vi "H5Sextent_copy.vi"(6 "error in (no error)":errorcluster, 8 "HDF5 Dest Space Ref":T1, 9 "HDF5 Source Space Ref":T1) -> (0 "error out":errorcluster, 2 "HDF5 Dest Space Ref out":T1, 3 "HDF5 Source Ref out":T1)   [LabVIEW 2017]
doc: "Copies the extent of a dataspace."
uses:
  <vilib>/UPVI/lvhdf5/library.llb/HDF5 Ref.ctl
  <vilib>/UPVI/lvhdf5/hdf5.dll
panel:
  # "LVHDF5 Toolkit\nCopyright (c) 2005-2013 by Jason D. Sommerville\nCopyright (c) 2014 by UPVI, LLC.\n\nThis use and distribution of this file is governed by the terms found in \nLICENSE.txt distributed with this toolkit and installed at\n <user.lib>\\_lvhdf5\\LICENSE.txt"
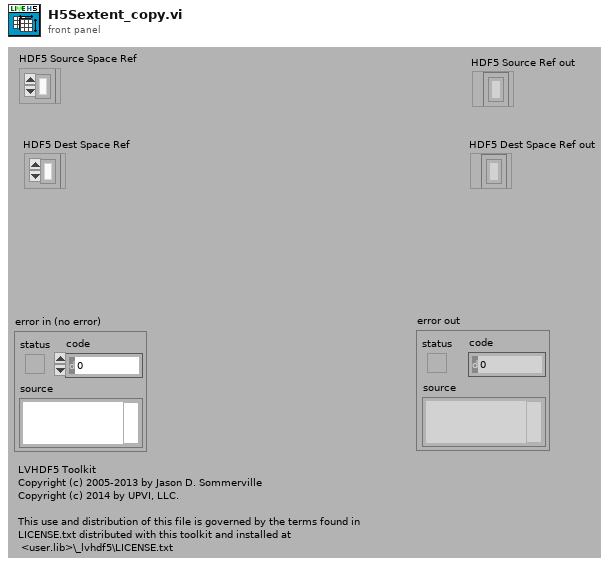
[diagram p1: front panel]
types:
  T1 = typedef "HDF5 Ref.ctl" = refnum<k1>
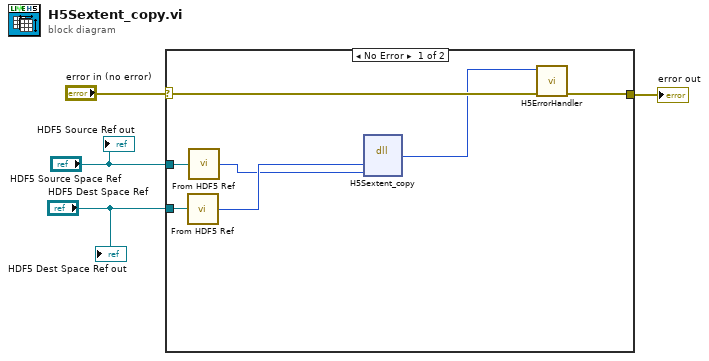
[diagram p0: block diagram]
diagram:
  n1 = case shown="No Error" "error in (no error)" {
    selector: "error in (no error)" -> [w11 w12]
    tunnel: [w10 w12] -> w3
    tunnel: "HDF5 Source Space Ref" -> [w9 _]
    tunnel: "HDF5 Dest Space Ref" -> [w7 _]
    frame No Error {
      n2 = call <vilib>:"From HDF5 Ref.vi"("HDF5 Ref"=w7) -> ("I32"=w6:i32)
      n3 = call <vilib>:"From HDF5 Ref.vi"("HDF5 Ref"=w9) -> ("I32"=w5:i32)
      n4 = dll-call lib="C:/Program Files/National Instruments/LabVIEW 2017/vi.lib/UPVI/lvhdf5/hdf5.dll" fn="H5Sextent_copy"("dest_space_id"=w6, "source_space_id"=w5) -> (w8:i32)  [unwired: 5 in, 2 out]
      n5 = call <vilib>:"H5ErrorHandler.vi"("error in (no error)"=w11, "herr_t"=w8) -> ("error out"=w10:errorcluster)  [unwired: 3 in, 4 out]
    }
    frame Error {
    }
  }
  "error out" <- w3
  "HDF5 Source Ref out" <- "HDF5 Source Space Ref"
  "HDF5 Dest Space Ref out" <- "HDF5 Dest Space Ref"
